vi "ODPLiveSim.vi"() -> ()   [LabVIEW 2018]
uses:
  State.ctl
  Constraints.ctl
  <extravilib>/ChannelInstances/Tag-class'TrapezoidalProfile'/Read With Abort.vi
  <extravilib>/ChannelInstances/Tag-class'TrapezoidalProfile'/Write With Abort.vi
  <extravilib>/ChannelInstances/Tag-class'TrapezoidalProfile'/Instantiate.vi
  <extravilib>/ChannelInstances/Tag-class'TrapezoidalProfile'/EndpointRead.vi
  <extravilib>/ChannelInstances/Tag-class'TrapezoidalProfile'/Endpoint.vi
  TrapezoidalProfile.lvclass
  <extravilib>/ChannelInstances/Tag-class'TrapezoidalProfile'.lvlib
panel:
  out "Is Finished?":bool
  in  "Constraints":T1={"Max Velocity"=10.0, "Max Accel"=15.0}
  out "Position":dbl(slide) scale=0.0..8.0
  out "Waveform Chart":T2(graph)
  out "Output":T3
  in  "Position Setpoint":dbl(slide) scale=0.0..8.0
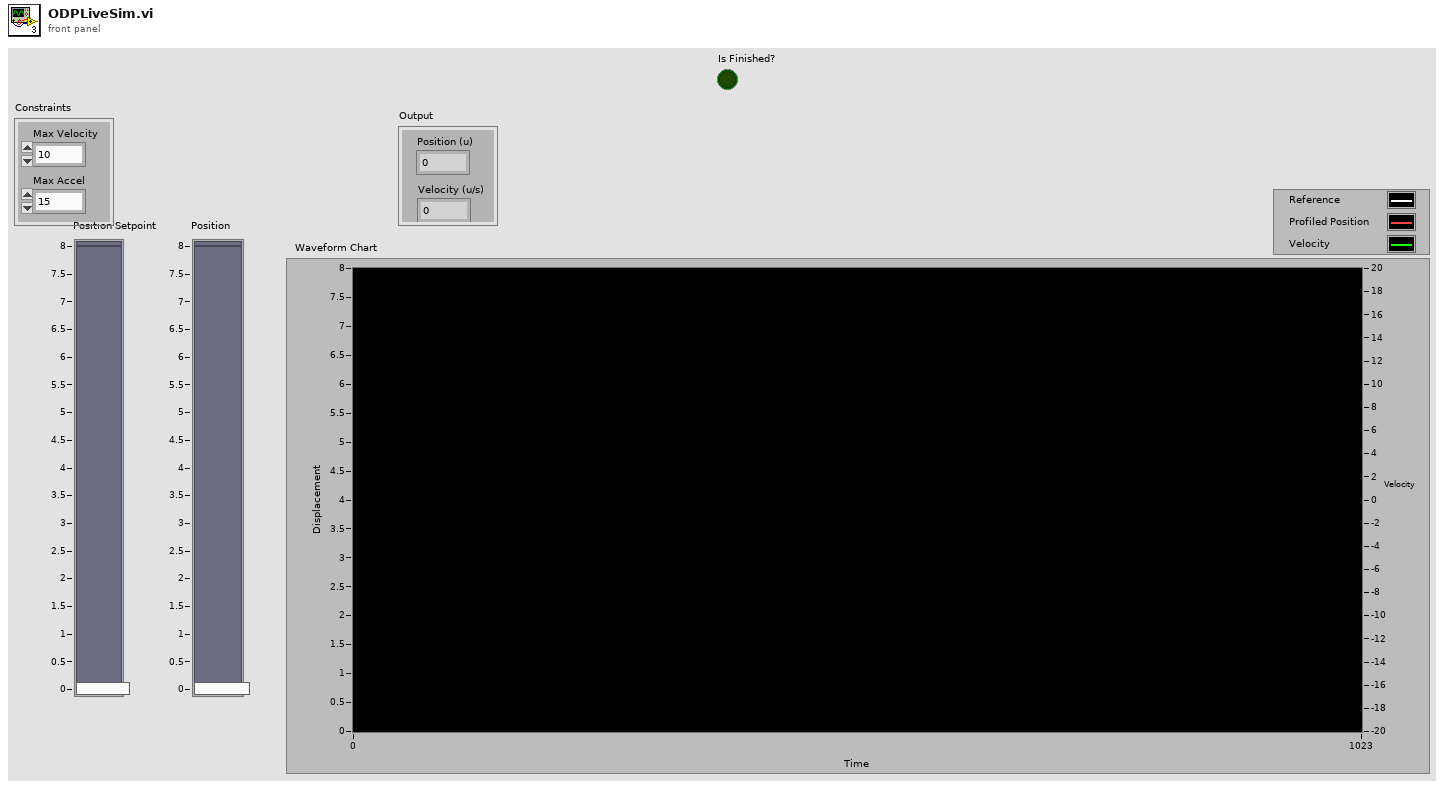
[diagram p1: front panel]
types:
  T1 = typedef "TrapezoidalProfile.lvclass/Constraints.ctl" = cluster{"Max Velocity":dbl, "Max Accel":dbl}
  T2 = cluster{"Position Setpoint":dbl, "Position (u)":dbl, "Velocity (u/s)":dbl}
  T3 = typedef "TrapezoidalProfile.lvclass/State.ctl" = cluster{"Position (u)":dbl, "Velocity (u/s)":dbl}
  T4 = typedef "Tag-class'TrapezoidalProfile'.lvlib/))Channel.ctl" = refnum<queue>
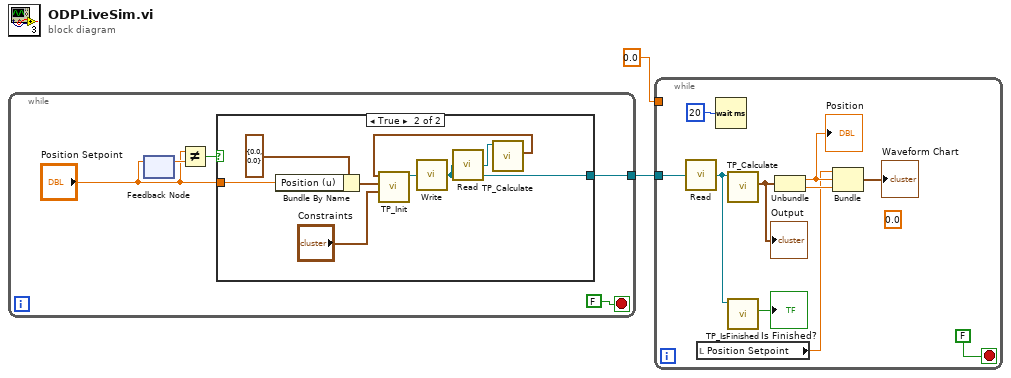
[diagram p0: block diagram]
diagram:
  n1 = while {
    tunnel: [w4] -> w1
    stop <- FALSE stop-if-true
    n2 = feedback-in #1("Position Setpoint") -> ()
    n3 = feedback #1() -> (w7:dbl)  [unwired: 1 in]
    n4 = Not Equal?(x="Position Setpoint", y=w7) -> (x != y?=w6:bool)
    n5 = case shown="True" w6 {
      tunnel: "Position Setpoint" -> [_ w9]
      tunnel: [_ w11] -> w4
      frame False {
      }
      frame True {
        n6 = Bundle By Name(cluster=T3 {"Position (u)"=0.0, "Velocity (u/s)"=0.0} ("Output"), "Position (u)"=w9) -> (w13:T3)
        n7 = call "TP_Init.vi"("Constraints"="Constraints", "Unprofiled Goal"=w13, "Initial"=w15) -> ("TrapezoidalProfile out"=w8:refnum<class "TrapezoidalProfile.lvclass">)  [unwired: 7 in, 1 out]
        n8 = call <extravilib>:"Write.vi"("element"=w8) -> ("channel"=w11:T4)  [unwired: 1 out]
        n9 = call <extravilib>:"Read.vi"("channel"=w11) -> ("element"=w12:refnum<class "TrapezoidalProfile.lvclass">)  [unwired: 1 in, 1 out]
        n10 = call "TP_Calculate.vi"("TrapezoidalProfile in"=w12) -> ("Output"=w15:T3)  [unwired: 8 in, 2 out]
      }
    }
  }
  n11 = while {
    tunnel: 0.0 ("Position Setpoint") -> [_]
    tunnel: w1 -> [w19]
    stop <- FALSE stop-if-true
    (unwired) 0.0
    n12 = call <extravilib>:"Read.vi"("channel"=w19) -> ("element"=w16:refnum<class "TrapezoidalProfile.lvclass">)  [unwired: 1 in, 1 out]
    n13 = local read "Position Setpoint"() -> (w17:dbl)
    n14 = Wait (ms)(milliseconds to wait=u32 20) -> ()  [unwired: 1 out]
    n15 = call "TP_Calculate.vi"("TrapezoidalProfile in"=w16) -> ("Output"=w21:T3)  [unwired: 8 in, 2 out]
    "Output" <- w21
    n16 = call "TP_IsFinished.vi"("TrapezoidalProfile in"=w16) -> ("Is Finished?"=→"Is Finished?":bool)  [unwired: 8 in, 2 out]
    n17 = Unbundle(w21) -> ("Position (u)"=w22:dbl, "Velocity (u/s)"=w25:dbl)
    "Position" <- w22
    n18 = Bundle("Position Setpoint"=w17, "Position (u)"=w22, "Velocity (u/s)"=w25) -> (→"Waveform Chart":T2)  [unwired: 1 in]
  }
